vi "initialise.vi"(8 "error in (no error)":errorcluster, 11 "RoiGeneric in":refnum<class "RoiGeneric.lvclass">) -> (0 "error out":errorcluster, 3 "RoiGeneric out":refnum<class "RoiGeneric.lvclass">)   [LabVIEW 2010, in "RoiGeneric.lvclass"]
uses:
  RoiGeneric.lvclass
  RoiGeneric.lvclass/RoiGeneric.ctl
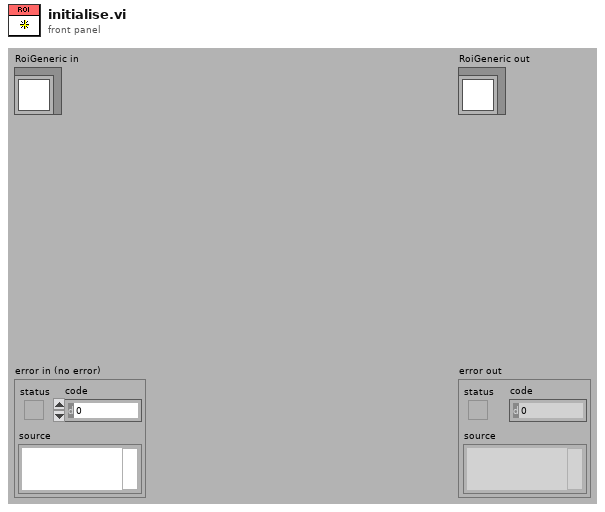
[diagram p1: front panel]
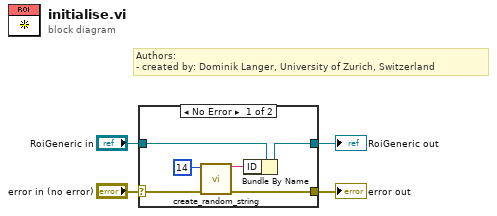
[diagram p0: block diagram]
diagram:
  # "Authors: \n- created by: Dominik Langer, University of Zurich, Switzerland"
  n1 = case shown="No Error" "error in (no error)" {
    selector: "error in (no error)" -> [w7 w12]
    tunnel: [w6 w12] -> w3
    tunnel: [w9 w11] -> w1
    tunnel: "RoiGeneric in" -> [w10 w11]
    frame No Error {
      n2 = call "create_random_string.vi"("error in (no error)"=w7, "length"=14) -> ("error out"=w6:errorcluster, "random string"=w8:string)  [unwired: 8 in]
      n3 = Bundle By Name(cluster=w10, "ID"=w8) -> (w9:refnum<class "RoiGeneric.lvclass">)
    }
    frame Error {
    }
  }
  "error out" <- w3
  "RoiGeneric out" <- w1
